vi "trafic light.vi"() -> ()   [LabVIEW 2021]
panel:
  out "Time":dbl
  out "Green":bool
  in  "Green time":dbl
  in  "Yellow time":dbl
  in  "Red time":dbl
  in  "?":bool
  out "Yellow":bool
  out "Red":bool
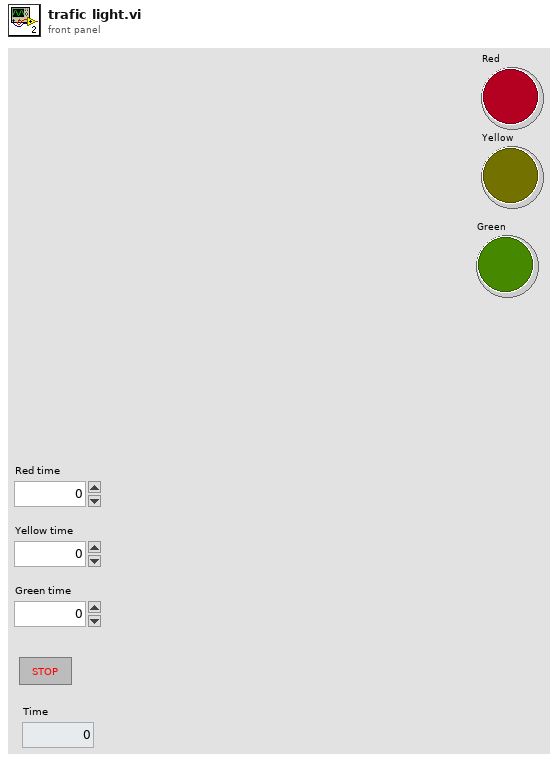
[diagram p1: front panel]
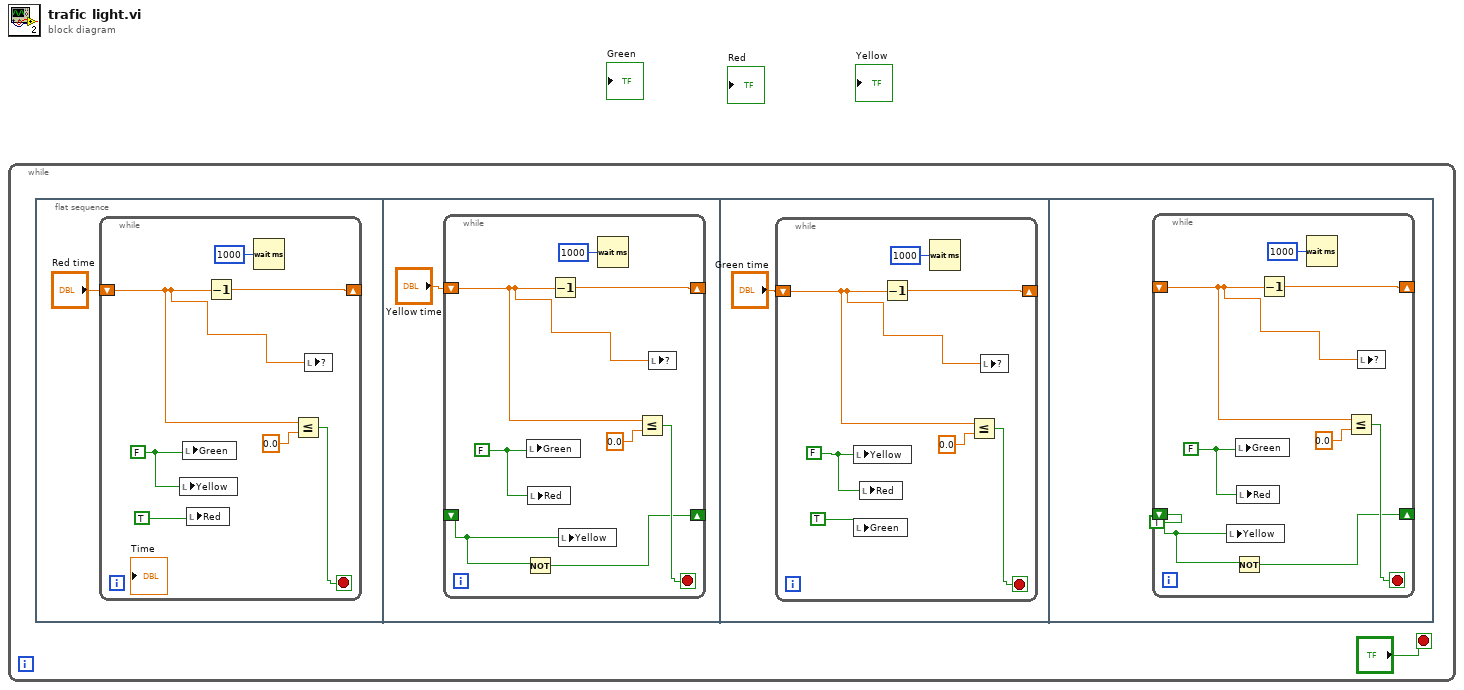
[diagram p0: block diagram]
diagram:
  n1 = while {
    stop <- "?" stop-if-true
    n2 = flat-sequence {
      frame #0 {
        n3 = while {
          shift-right: [w7] -> _
          shift-left: "Red time" -> [w6]
          stop <- w4 stop-if-true
          w9 = FALSE
          n4 = local write "Yellow"(w9) -> ()
          n5 = local write "Green"(w9) -> ()
          n6 = local write "Red"(TRUE) -> ()
          n7 = Decrement(x=w6) -> (x-1=w7:dbl)
          n8 = Wait (ms)(milliseconds to wait=u32 1000) -> ()  [unwired: 1 out]
          n9 = Less Or Equal?(x=w6, y=0.0) -> (x <= y?=w4:bool)
          n10 = local write item#-1(w6) -> ()
        }
      }
      frame #1 {
        n11 = while {
          shift-right: [w18] -> _
          shift-left: "Yellow time" -> [w17]
          shift-right: [w12] -> _
          shift-left: _ -> [w11]
          stop <- w15 stop-if-true
          w13 = FALSE
          n12 = Not(x=w11) -> (.not. x?=w12:bool)
          n13 = local write "Green"(w13) -> ()
          n14 = local write "Red"(w13) -> ()
          n15 = Decrement(x=w17) -> (x-1=w18:dbl)
          n16 = local write "Yellow"(w11) -> ()
          n17 = Wait (ms)(milliseconds to wait=u32 1000) -> ()  [unwired: 1 out]
          n18 = Less Or Equal?(x=w17, y=0.0) -> (x <= y?=w15:bool)
          n19 = local write item#-1(w17) -> ()
        }
      }
      frame #2 {
        n20 = while {
          shift-right: [w26] -> _
          shift-left: "Green time" -> [w25]
          stop <- w23 stop-if-true
          w21 = FALSE
          n21 = local write "Yellow"(w21) -> ()
          n22 = local write "Green"(TRUE) -> ()
          n23 = local write "Red"(w21) -> ()
          n24 = Decrement(x=w25) -> (x-1=w26:dbl)
          n25 = Wait (ms)(milliseconds to wait=u32 1000) -> ()  [unwired: 1 out]
          n26 = Less Or Equal?(x=w25, y=0.0) -> (x <= y?=w23:bool)
          n27 = local write item#-1(w25) -> ()
        }
      }
      frame #3 {
        n28 = while {
          shift-right: [w36] -> _
          shift-left: [w35] -> w28
          shift-right: [w30] -> _
          shift-left: TRUE -> [w29]
          stop <- w33 stop-if-true
          w31 = FALSE
          n29 = local write "Yellow"(w29) -> ()
          n30 = Not(x=w29) -> (.not. x?=w30:bool)
          n31 = local write "Green"(w31) -> ()
          n32 = local write "Red"(w31) -> ()
          n33 = Decrement(x=w35) -> (x-1=w36:dbl)
          n34 = Wait (ms)(milliseconds to wait=u32 1000) -> ()  [unwired: 1 out]
          n35 = Less Or Equal?(x=w35, y=0.0) -> (x <= y?=w33:bool)
          n36 = local write item#-1(w35) -> ()
        }
      }
    }
  }
